vi "Actor Core.vi"(8 "error in":errorcluster caption="错误输入", 11 "ParentActor in":refnum<class "ParentActor.lvclass"> caption="操作者输入") -> (0 "error out":errorcluster caption="错误输出", 3 "Actor out":refnum<class "Actor.lvclass"> caption="操作者输出")   [LabVIEW 2014, in "UnitTest.lvlib" / "ParentActor.lvclass"]
doc: "(<B>文件名</B>：Actor Framework.lvlib:Actor.lvclass:Actor Core.vi)\n\n接收发送至操作者的消息，响应消息并处理可能导致操作者关闭的错误。\n\n子孙类重写该VI，使操作者完成特定的任务。使用调用父方法节点实现重写。"
uses:
  ParentActor.lvclass
  <vilib>/ActorFramework/Actor/Actor.lvclass
  MiddleSlaveActor/MiddleSlaveActor.lvclass
  MiddleMasterActor/MiddleMasterActor.lvclass
  <vilib>/ActorFramework/Actor/Actor.lvclass/Actor.ctl
  <vilib>/ActorFramework/Message Enqueuer/Message Enqueuer.lvclass/Message Enqueuer.ctl
  <vilib>/ActorFramework/Message Enqueuer/Init from Existing Queue.vi
  <vilib>/ActorFramework/Message Enqueuer/Enqueue.vi
  <vilib>/ActorFramework/Message Priority Queue/Priority Enqueue.vi
  <vilib>/ActorFramework/Message Enqueuer/Message Enqueuer.lvclass
  <vilib>/ActorFramework/Stop Msg/Stop Msg.lvclass
  Wrapper_lib/zsActor/ActorWrapper.lvclass
types:
  T1 = enum16{"OpenSlaveActor", "Idle", "StopSlaveActor"}
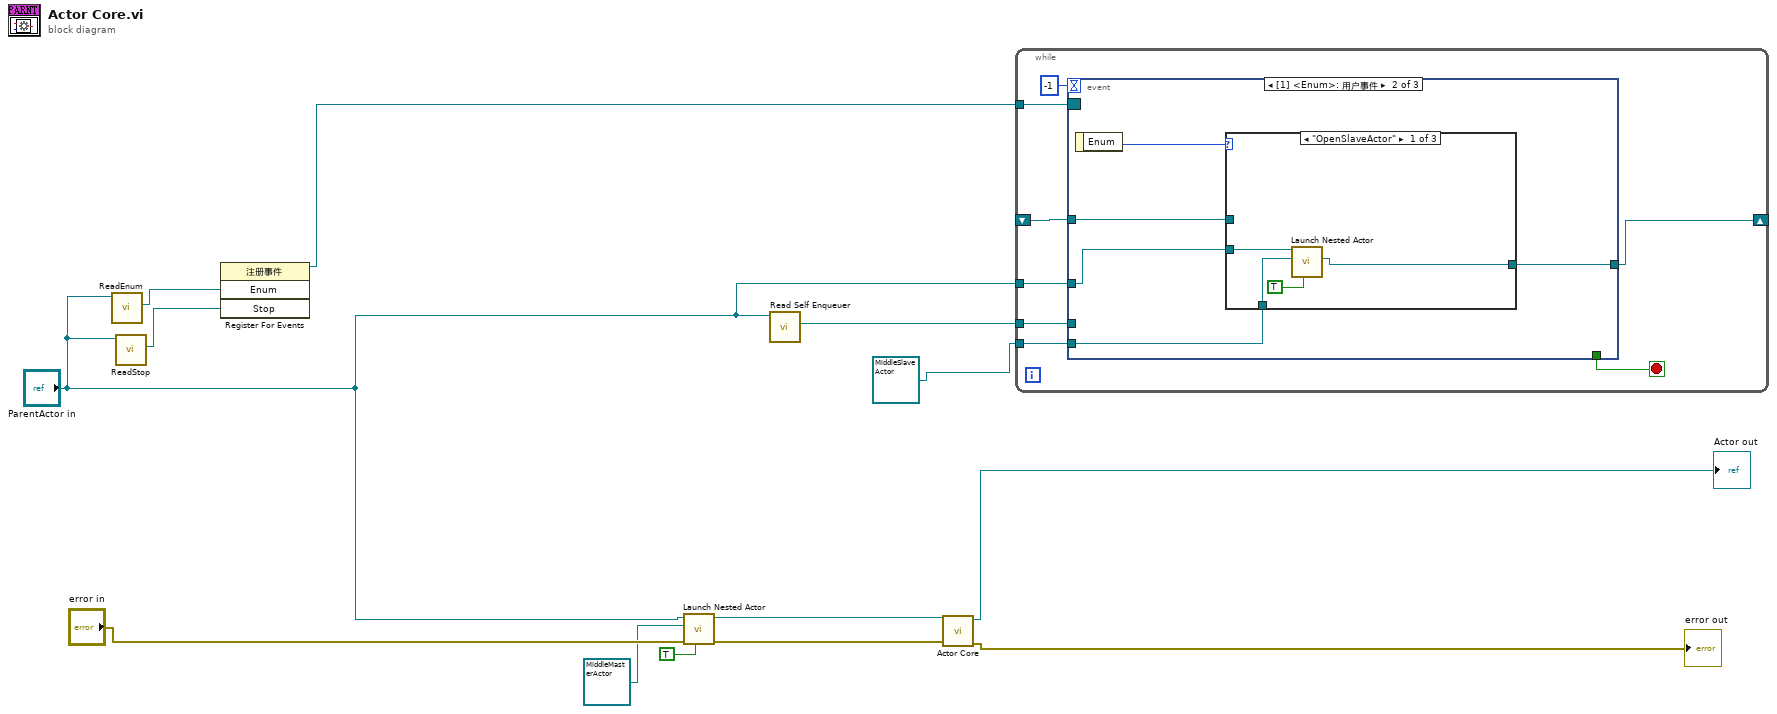
[diagram p0: block diagram]
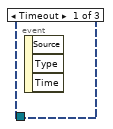
[diagram p2: hidden frame]
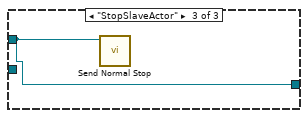
[diagram p4: hidden frame]
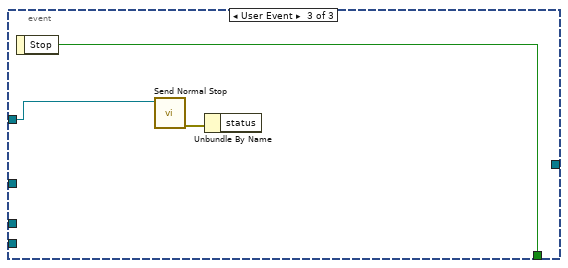
[diagram p5: hidden frame]
diagram:
  n1 = call-dynamic "ReadEnum.vi"("zsActor输入"="ParentActor in") -> ("Enum"=w8:refnum<user-event>)  [unwired: 8 in, 2 out]
  n2 = call-dynamic "ReadStop.vi"("zsActor输入"="ParentActor in") -> ("Stop"=w7:refnum<user-event>)  [unwired: 8 in, 2 out]
  n3 = register-events(w8, w7) -> (reference out=w10:refnum<event-registration>)  [unwired: 2 in, 1 out]
  n4 = call <vilib>:"Launch Nested Actor.vi"("Open Actor Core front panel? (F)"=TRUE, "error in (no error)"="error in", "Nested Actor"=refnum<class "MiddleMasterActor.lvclass"> refnum ("TestActors.lvlib:MiddleMasterActor.lvclass"), "Caller Actor in"="ParentActor in") -> ("error out"=w2:errorcluster, "Caller Actor out"=w3:refnum<class "ParentActor.lvclass">)  [unwired: 5 in, 1 out]
  n5 = call <vilib>:"Read Self Enqueuer.vi"("Actor"="ParentActor in") -> ("Self Enqueuer"=w11:refnum<class "Message Enqueuer.lvclass">)  [unwired: 10 in]
  n6 = call-parent "Actor Core.vi"("error in"=w2, "Actor in"=w3) -> ("error out"=→"error out":errorcluster, "Actor out"=→"Actor out":refnum<class "Actor.lvclass">)  [unwired: 8 in]
  n7 = while {
    tunnel: w11 -> [w18]
    tunnel: "ParentActor in" -> [w21]
    tunnel: refnum<class "MiddleSlaveActor.lvclass"> refnum ("TestActors.lvlib:MiddleSlaveActor.lvclass") -> [w20]
    shift-right: [w19] -> _
    shift-left: _ -> [w16]
    tunnel: w10 -> [w15]
    stop <- w14 stop-if-true
    n8 = event shown="[1] <Enum>: 用户事件" {
      selector: w15 -> [_ _ _]
      dyn-events: _ -> [_ _ _]
      timeout: -1 -> [_ _ _]
      tunnel: w21 -> [_ w25 _]
      tunnel: w20 -> [_ w26 _]
      tunnel: [_ w24 _] -> w19
      tunnel: w18 -> [_ _ _]
      tunnel: w16 -> [_ w23 w34]
      tunnel: [_ _ w35] -> w14
      event Timeout {
        n9 = event-data() -> ()  [unwired: 1 in, 3 out]
      }
      event User Event {
        n10 = event-data() -> ("Enum"=w22:T1)  [unwired: 1 in]
        n11 = case shown="\"OpenSlaveActor\"" w22 {
          tunnel: w26 -> [w30 _ _]
          tunnel: w25 -> [w29 _ _]
          tunnel: [w27 w31 w32] -> w24
          tunnel: w23 -> [_ w31 w32]
          frame "OpenSlaveActor" {
            n12 = call <vilib>:"Launch Nested Actor.vi"("Open Actor Core front panel? (F)"=TRUE, "Nested Actor"=w30, "Caller Actor in"=w29) -> ("Nested Actor's Enqueuer"=w27:refnum<class "Message Enqueuer.lvclass">)  [unwired: 6 in, 2 out]
          }
          frame "Idle", Default {
          }
          frame "StopSlaveActor" {
            n13 = call <vilib>:"Send Normal Stop.vi"("Message Enqueuer"=w32) -> ()  [unwired: 10 in, 1 out]
          }
        }
      }
      event User Event {
        n14 = event-data() -> ("Stop"=w35:bool)  [unwired: 1 in]
        n15 = call <vilib>:"Send Normal Stop.vi"("Message Enqueuer"=w34) -> ("error out"=w33:errorcluster)  [unwired: 10 in]
        n16 = Unbundle By Name(w33) -> ()  [unwired: 1 out]
      }
    }
  }
